vi "ma_sml_Window Frequency Response (first derivative, double).vi"(1 "N (window length)":i32, 2 "window":u16(ring) items=["Rectangle"=0, "Hanning"=1, "Hamming"=2, "Blackman-Harris"=3, "Exact Blackman"=4, "Blackman"=5, "Flat Top"=6, "4 Term B-Harris "=7, "7 Term B-Harris"=8, "Low Sidelobe"=9, "Blackman Nuttall"=11, "Triangle"=30, "Bartlett-Hanning"=31, "Bohman"=32, "Parzen"=33, "Welch"=34, "Kaiser"=60, "Dolph-Chebyshev"=61, "Gaussian"=62], 3 "f(normalized)":dbl format="%.5e") -> (0 "H'(f)":dbl format="%.5e")   [LabVIEW 2020, in "NI_MAPro.lvlib"]
uses:
  NI_MAPro.lvlib
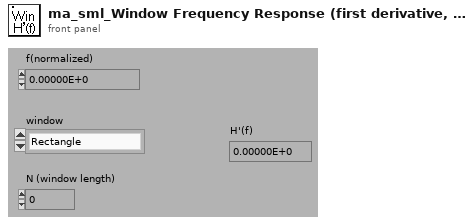
[diagram p1: front panel]
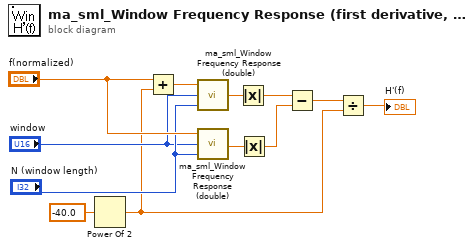
[diagram p0: block diagram]
diagram:
  n1 = Power Of 2(x=-40.0) -> (2^x=w2:dbl)
  n2 = Add(x="f(normalized)", y=w2) -> (x+y=w12:dbl)
  n3 = call "ma_sml_Window Frequency Response (double).vi"("N (window length)"="N (window length)", "window"="window", "f(normalized)"=w12) -> ("H(f)"=w7:cdb)
  n4 = call "ma_sml_Window Frequency Response (double).vi"("N (window length)"="N (window length)", "window"="window", "f(normalized)"="f(normalized)") -> ("H(f)"=w6:cdb)
  n5 = Absolute Value(x=w7) -> (abs(x)=w5:dbl)
  n6 = Absolute Value(x=w6) -> (abs(x)=w4:dbl)
  n7 = Subtract(x=w5, y=w4) -> (x-y=w3:dbl)
  n8 = Divide(x=w3, y=w2) -> (x/y=→"H'(f)":dbl)
